vi "Load Calibration Coefficients.vi"() -> (3 "Calibration Coefficients":T1[](array[typedef]) {"Elapsed Time" format="%<%H:%M:%S>t"; "Pump Flow Rate" format="%0d"; "Number of Zeroes" format="%0d"; "V2C" format="%0d"; "C2V" format="%0d"; "duration" format="%<%H:%M:%S>t"; "DAC" format="%03x"; "mI" format="%.3g"; "V_(RA,15mA)" format="%0.4f"; "V_(RA,5mA)" format="%0.4f"; "Chamber Temp" format="%.1f"; "Humidity" format="%.1f"})   [LabVIEW 2016]
uses:
  Controls/Calibration Coefficients.ctl
  Miscellaneous/Globals.vi
panel:
  out "Numeric":i32
  out "size(s)":i32[](array[numeric])
  out "Fini":string
  out "Spreadsheet":string[][](array[string])
  in  "Calfile":path=path "~last_calibration.csv"
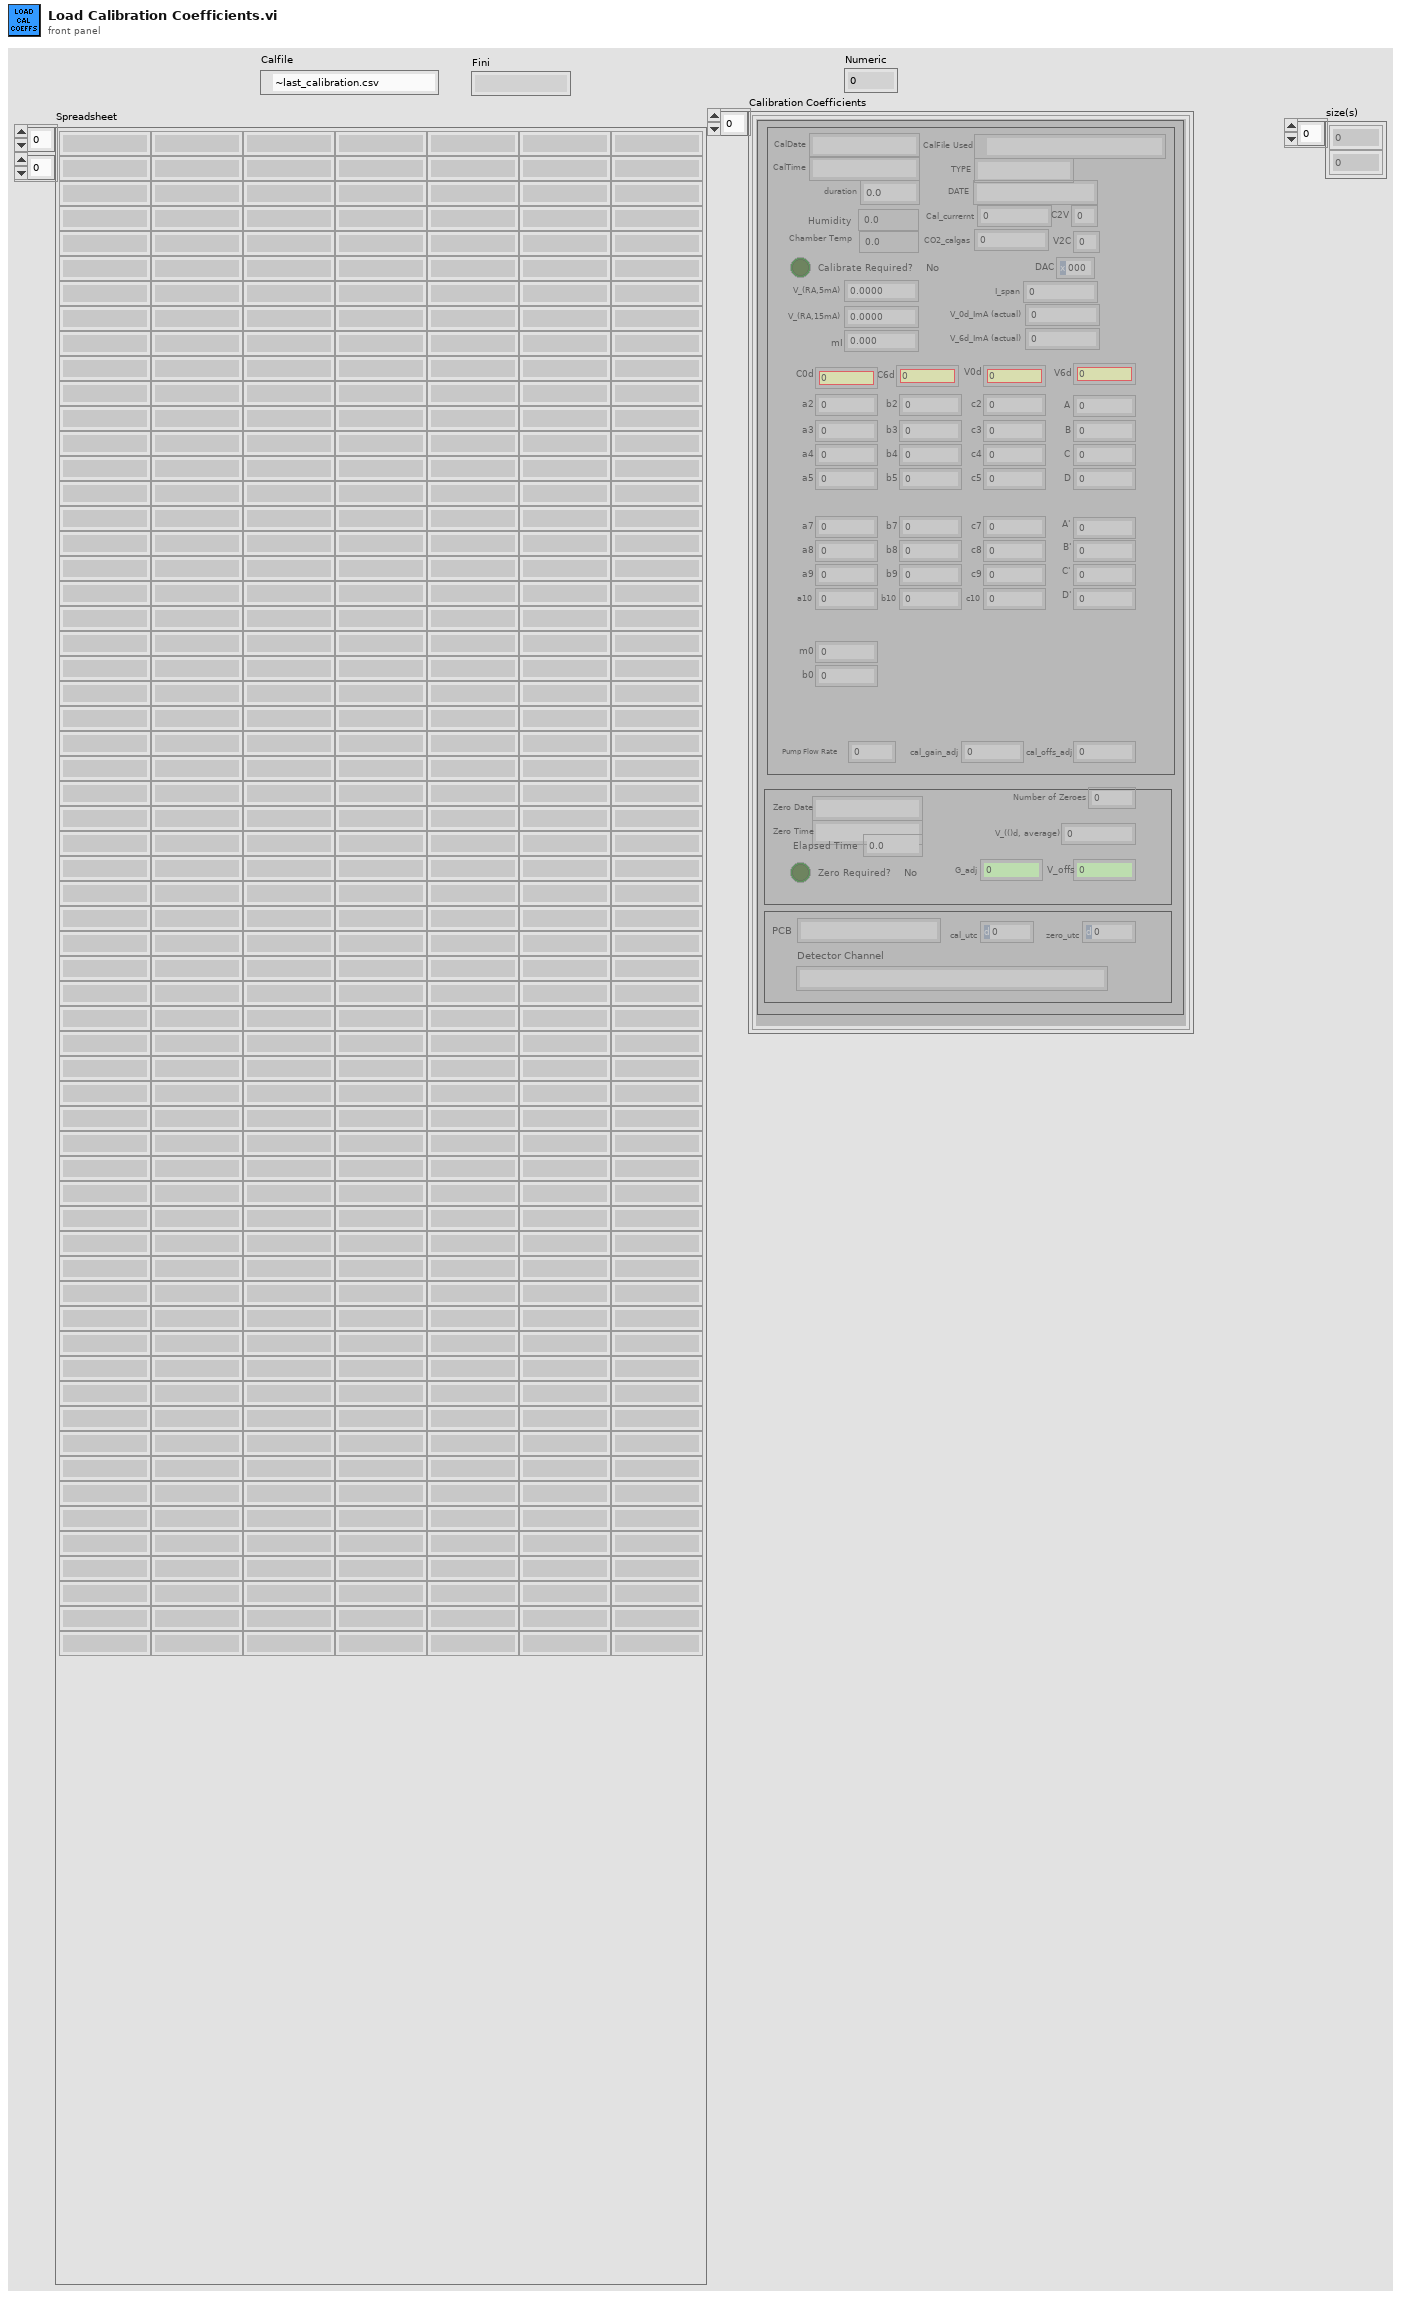
[diagram p1: front panel]
types:
  T1 = typedef "Calibration Coefficients.ctl" = cluster{"CalFile Used":path, "TYPE":string, "DATE":string, "Humidity":sgl, "Chamber Temp":dbl, "CO2_calgas":dbl, "V_(RA,5mA)":dbl, "V_(RA,15mA)":dbl, "mI":dbl, "V_0d_ImA (actual)":dbl, "V_6d_ImA (actual)":dbl, "I_span":dbl, "DAC":u16, "A":dbl, "B":dbl, "C":dbl, "D":dbl, "V6d":dbl, "A'":dbl, "B'":dbl, "C'":dbl, "D'":dbl, "V0d":dbl, "CalDate":string, "CalTime":string, "duration":dbl, "Detector Channel":string, "a2":dbl, "a3":dbl, "a4":dbl, "a5":dbl, "b2":dbl, "c2":dbl, "b3":dbl, "c3":dbl, "b4":dbl, "c4":dbl, "b5":dbl, "c5":dbl, "a7":dbl, "a8":dbl, "a9":dbl, "a10":dbl, "b7":dbl, "b8":dbl, "b9":dbl, "b10":dbl, "c7":dbl, "c8":dbl, "c9":dbl, "c10":dbl, "cal_offs_adj":dbl, "cal_gain_adj":dbl, "C6d":dbl, "C0d":dbl, "Cal_currernt":dbl, "C2V":u16, "V2C":u16, "Zero Date":string, "Zero Time":string, "Number of Zeroes":u16, "V_(()d, average)":dbl, "V_offs ":dbl, "G_adj":dbl, "Pump Flow Rate":u16, "Zero Required? ":bool, "Calibrate Required?":bool, "cal_utc":dbl, "zero_utc":dbl, "Elapsed Time":dbl, "PCB":string, "m0":dbl, "b0":dbl}
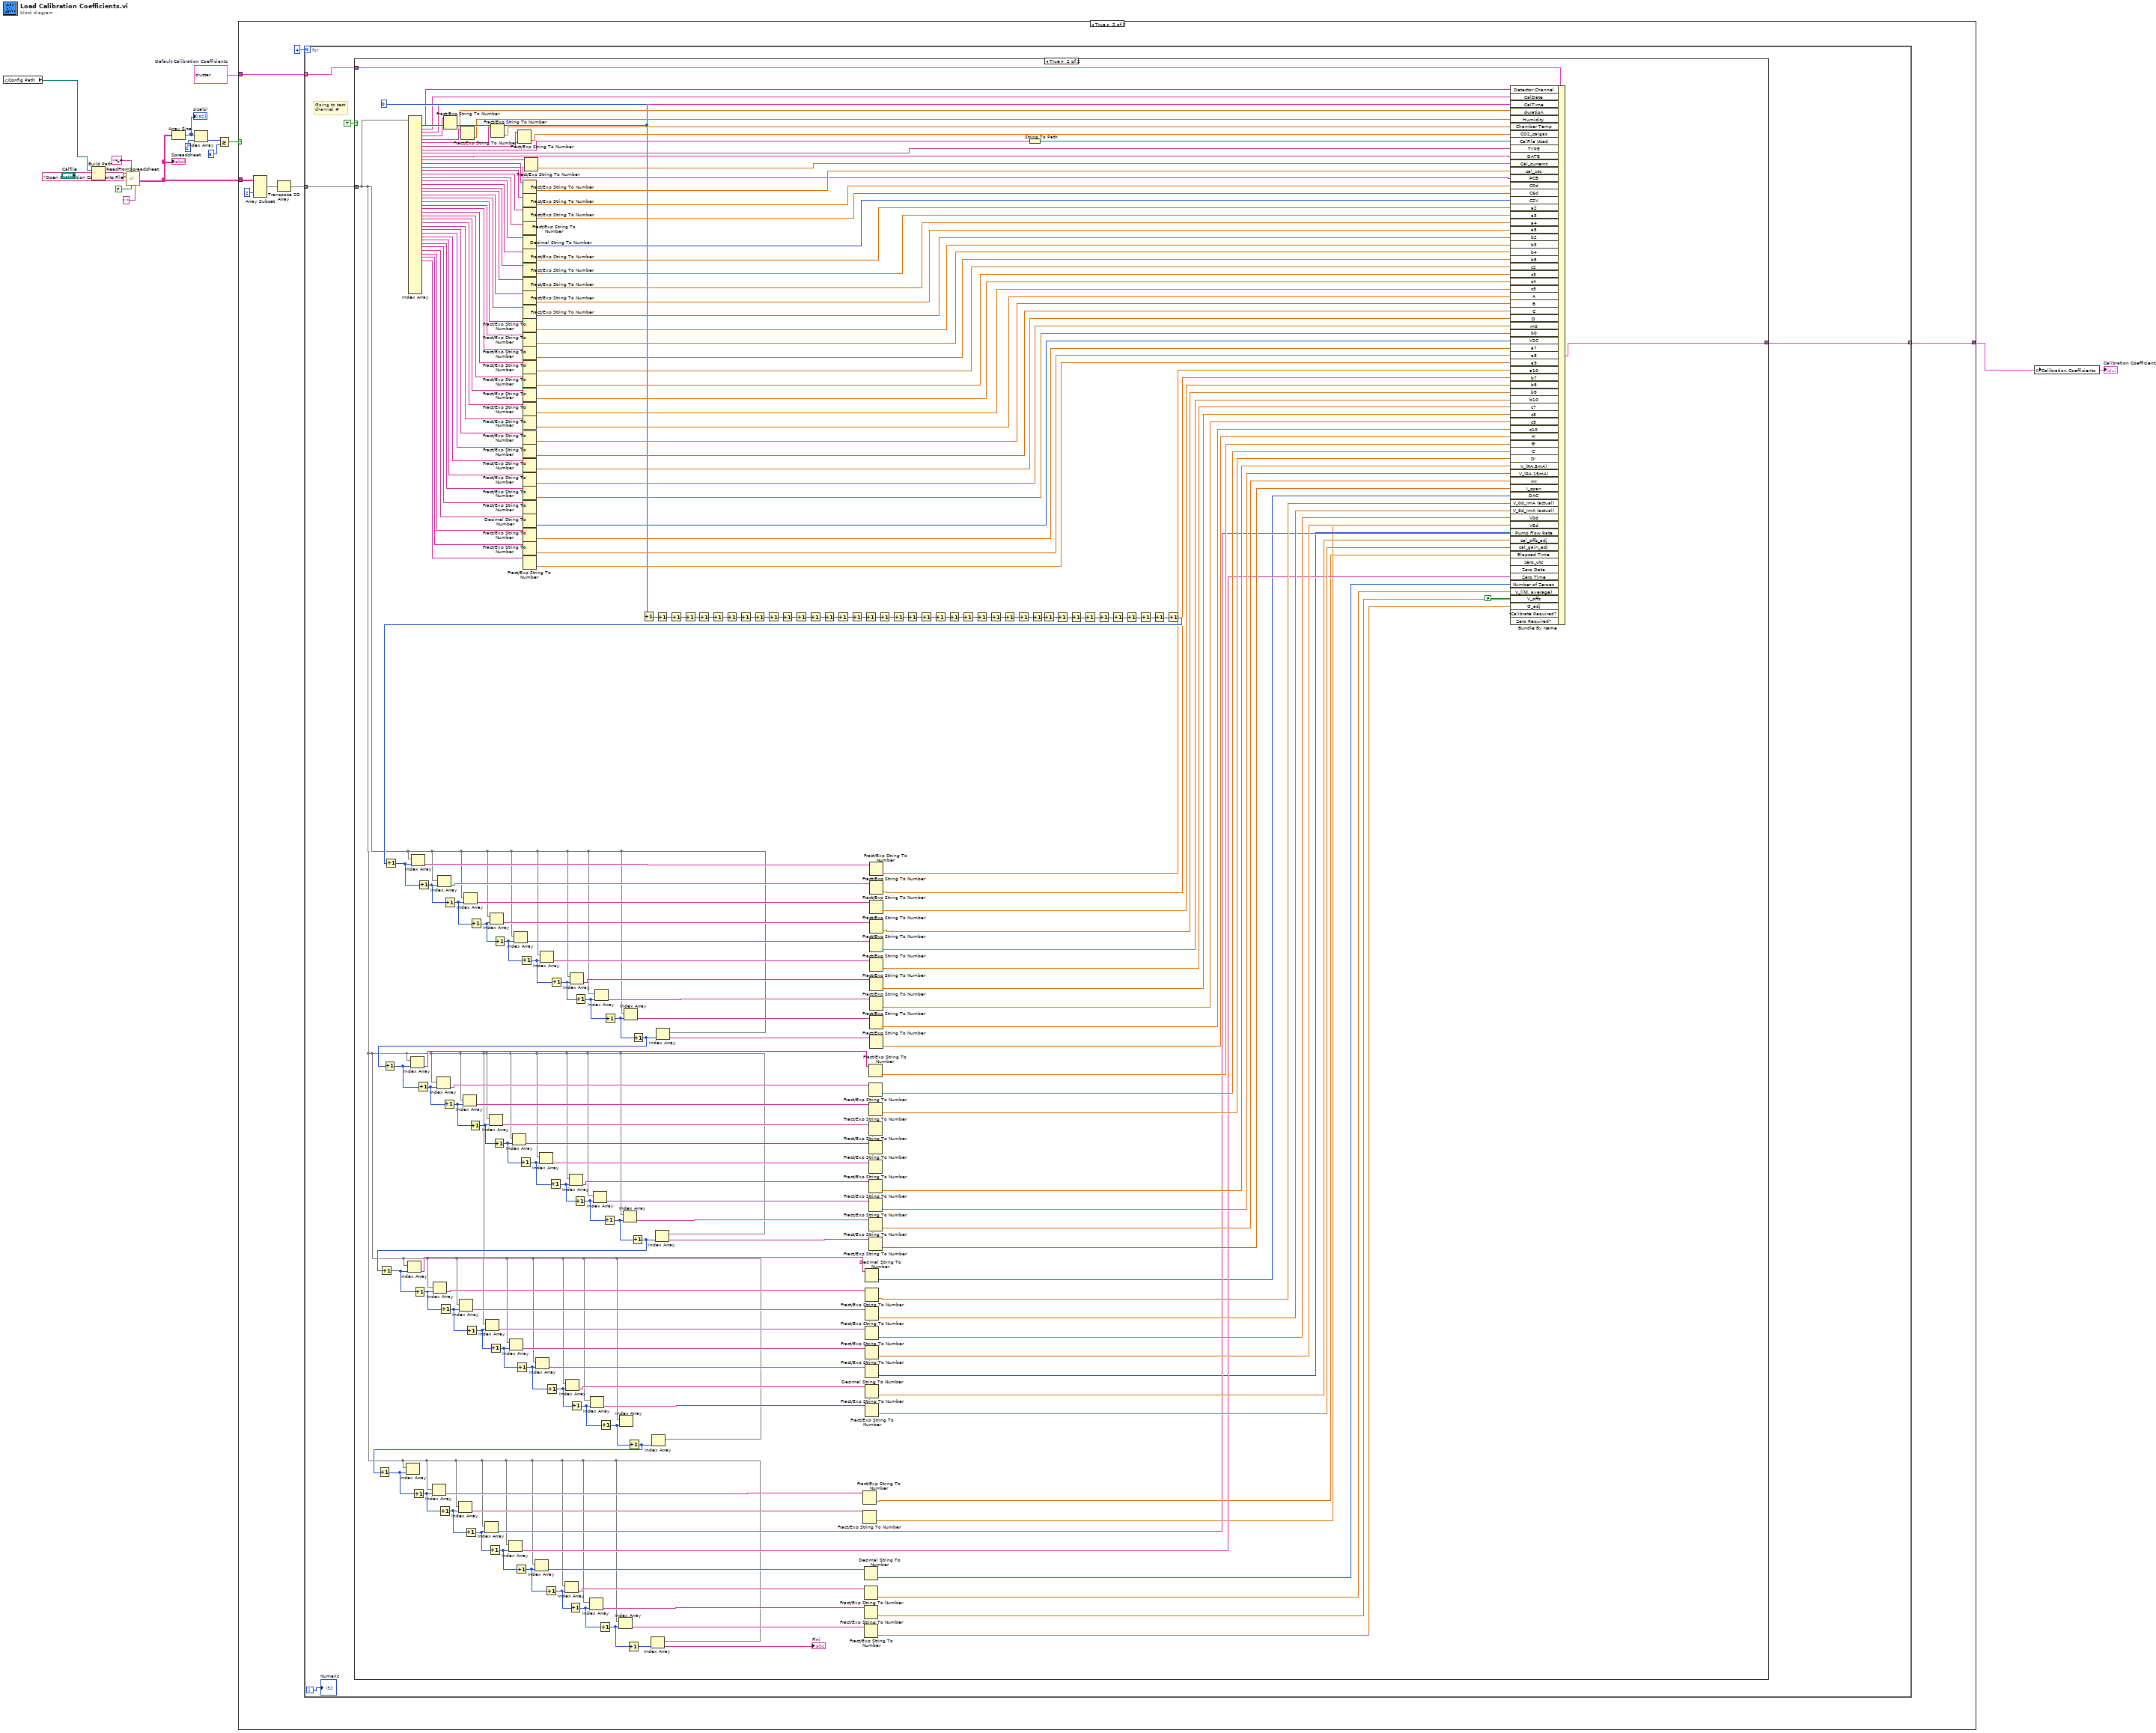
[diagram p0: block diagram]
diagram:
  w4 = T1[] [{"CalFile Used"=path "C:/Users/Bench2/Dropbox/PAHS Public/AK Temp/Coefficients/AE_coefficents.CSV", "TYPE"="CalCoeff", "DATE"="[04-07-15]&[04-16-15]", "Humidity"=114.68759, "Chamber Temp"=20.714597, "CO2_calgas"=6.0, "V_(RA,5mA)"=0.52354, "V_(RA,15mA)"=1.619069, "mI"=109.552915, "V_0d_ImA (actual)"=1.442862, "V_6d_ImA (actual)"=4.943226, "I_span"=0.0132, "DAC"=126, "A"=0.008886, "B"=-0.182423, "C"=1.620623, "D"=1.075523, "V6d"=6.151482, "A'"=0.029909, "B'"=-0.16462, "C'"=0.985378, "D'"=-0.927836, "V0d"=1.188075, "CalDate"="6/2/2015", "CalTime"="4:50:14 PM", "duration"=214.0, "Detector Channel"="1", "a2"=1.6e-05, "a3"=-0.000231, "a4"=0.000552, "a5"=-0.001022, "b2"=-0.001316, "c2"=0.029462, "b3"=0.021946, "c3"=-0.537873, "b4"=-0.098377, "c4"=3.421543, "b5"=0.038523, "c5"=0.716135, "a7"=2e-05, "a8"=0.000362, "a9"=0.00167, "a10"=-0.001204, "b7"=-0.000903, "b8"=-0.00141, "b9"=-0.087565, "b10"=0.06077, "c7"=0.040003, "c8"=-0.29086, "c9"=2.082505, "c10"=-1.670048, "cal_offs_adj"=0.254787, "cal_gain_adj"=1.004082, "C6d"=5.866368, "C0d"=0.060659, "Cal_currernt"=8.0, "C2V"=4, "V2C"=4, "Zero Date"="6/2/2015", "Zero Time"="4:50:18 PM", "Number of Zeroes"=0, "V_(()d, average)"=1.442862, "V_offs "=0.254787, "G_adj"=1.004082, "Pump Flow Rate"=150, "Zero Required? "=FALSE, "Calibrate Required?"=FALSE, "cal_utc"=3516105014.176389, "zero_utc"=3516105018.776652, "Elapsed Time"=0.0, "PCB"="", "m0"=nan, "b0"=nan}, {"CalFile Used"=path "C:/Users/Bench2/Dropbox/PAHS Public/AK Temp/Coefficients/AE_coefficents.CSV", "TYPE"="CalCoeff", "DATE"="[04-07-15]&[04-16-15]", "Humidity"=114.68759, "Chamber Temp"=20.714597, "CO2_calgas"=6.0, "V_(RA,5mA)"=0.52354, "V_(RA,15mA)"=1.619069, "mI"=109.552915, "V_0d_ImA (actual)"=1.442862, "V_6d_ImA (actual)"=4.943226, "I_span"=0.0132, "DAC"=126, "A"=0.008886, "B"=-0.182423, "C"=1.620623, "D"=1.075523, "V6d"=6.151482, "A'"=0.029909, "B'"=-0.16462, "C'"=0.985378, "D'"=-0.927836, "V0d"=1.188075, "CalDate"="6/2/2015", "CalTime"="4:50:14 PM", "duration"=214.0, "Detector Channel"="2", "a2"=1.6e-05, "a3"=-0.000231, "a4"=0.000552, "a5"=-0.001022, "b2"=-0.001316, "c2"=0.029462, "b3"=0.021946, "c3"=-0.537873, "b4"=-0.098377, "c4"=3.421543, "b5"=0.038523, "c5"=0.716135, "a7"=2e-05, "a8"=0.000362, "a9"=0.00167, "a10"=-0.001204, "b7"=-0.000903, "b8"=-0.00141, "b9"=-0.087565, "b10"=0.06077, "c7"=0.040003, "c8"=-0.29086, "c9"=2.082505, "c10"=-1.670048, "cal_offs_adj"=0.254787, "cal_gain_adj"=1.004082, "C6d"=5.866368, "C0d"=0.060659, "Cal_currernt"=8.0, "C2V"=4, "V2C"=4, "Zero Date"="6/2/2015", "Zero Time"="4:50:18 PM", "Number of Zeroes"=0, "V_(()d, average)"=1.442862, "V_offs "=0.254787, "G_adj"=1.004082, "Pump Flow Rate"=150, "Zero Required? "=FALSE, "Calibrate Required?"=FALSE, "cal_utc"=3516105014.176389, "zero_utc"=3516105018.776652, "Elapsed Time"=0.0, "PCB"="", "m0"=nan, "b0"=nan}, {"CalFile Used"=path "C:/Users/Bench2/Dropbox/PAHS Public/AK Temp/Coefficients/AE_coefficents.CSV", "TYPE"="CalCoeff", "DATE"="[04-07-15]&[04-16-15]", "Humidity"=114.68759, "Chamber Temp"=20.714597, "CO2_calgas"=6.0, "V_(RA,5mA)"=0.52354, "V_(RA,15mA)"=1.619069, "mI"=109.552915, "V_0d_ImA (actual)"=1.442862, "V_6d_ImA (actual)"=4.943226, "I_span"=0.0132, "DAC"=126, "A"=0.008886, "B"=-0.182423, "C"=1.620623, "D"=1.075523, "V6d"=6.151482, "A'"=0.029909, "B'"=-0.16462, "C'"=0.985378, "D'"=-0.927836, "V0d"=1.188075, "CalDate"="6/2/2015", "CalTime"="4:50:14 PM", "duration"=214.0, "Detector Channel"="3", "a2"=1.6e-05, "a3"=-0.000231, "a4"=0.000552, "a5"=-0.001022, "b2"=-0.001316, "c2"=0.029462, "b3"=0.021946, "c3"=-0.537873, "b4"=-0.098377, "c4"=3.421543, "b5"=0.038523, "c5"=0.716135, "a7"=2e-05, "a8"=0.000362, "a9"=0.00167, "a10"=-0.001204, "b7"=-0.000903, "b8"=-0.00141, "b9"=-0.087565, "b10"=0.06077, "c7"=0.040003, "c8"=-0.29086, "c9"=2.082505, "c10"=-1.670048, "cal_offs_adj"=0.254787, "cal_gain_adj"=1.004082, "C6d"=5.866368, "C0d"=0.060659, "Cal_currernt"=8.0, "C2V"=4, "V2C"=4, "Zero Date"="6/2/2015", "Zero Time"="4:50:18 PM", "Number of Zeroes"=0, "V_(()d, average)"=1.442862, "V_offs "=0.254787, "G_adj"=1.004082, "Pump Flow Rate"=150, "Zero Required? "=FALSE, "Calibrate Required?"=FALSE, "cal_utc"=3516105014.176389, "zero_utc"=3516105018.776652, "Elapsed Time"=0.0, "PCB"="", "m0"=nan, "b0"=nan}, {"CalFile Used"=path "C:/Users/Bench2/Dropbox/PAHS Public/AK Temp/Coefficients/AE_coefficents.CSV", "TYPE"="CalCoeff", "DATE"="[04-07-15]&[04-16-15]", "Humidity"=114.68759, "Chamber Temp"=20.714597, "CO2_calgas"=6.0, "V_(RA,5mA)"=0.52354, "V_(RA,15mA)"=1.619069, "mI"=109.552915, "V_0d_ImA (actual)"=1.442862, "V_6d_ImA (actual)"=4.943226, "I_span"=0.0132, "DAC"=126, "A"=0.008886, "B"=-0.182423, "C"=1.620623, "D"=1.075523, "V6d"=6.151482, "A'"=0.029909, "B'"=-0.16462, "C'"=0.985378, "D'"=-0.927836, "V0d"=1.188075, "CalDate"="6/2/2015", "CalTime"="4:50:14 PM", "duration"=214.0, "Detector Channel"="4", "a2"=1.6e-05, "a3"=-0.000231, "a4"=0.000552, "a5"=-0.001022, "b2"=-0.001316, "c2"=0.029462, "b3"=0.021946, "c3"=-0.537873, "b4"=-0.098377, "c4"=3.421543, "b5"=0.038523, "c5"=0.716135, "a7"=2e-05, "a8"=0.000362, "a9"=0.00167, "a10"=-0.001204, "b7"=-0.000903, "b8"=-0.00141, "b9"=-0.087565, "b10"=0.06077, "c7"=0.040003, "c8"=-0.29086, "c9"=2.082505, "c10"=-1.670048, "cal_offs_adj"=0.254787, "cal_gain_adj"=1.004082, "C6d"=5.866368, "C0d"=0.060659, "Cal_currernt"=8.0, "C2V"=4, "V2C"=4, "Zero Date"="6/2/2015", "Zero Time"="4:50:18 PM", "Number of Zeroes"=0, "V_(()d, average)"=1.442862, "V_offs "=0.254787, "G_adj"=1.004082, "Pump Flow Rate"=150, "Zero Required? "=FALSE, "Calibrate Required?"=FALSE, "cal_utc"=3516105014.176389, "zero_utc"=3516105018.776652, "Elapsed Time"=0.0, "PCB"="", "m0"=nan, "b0"=nan}]  # Default Calibration Coefficients
  n1 = global read "Globals.vi" "Config Path"() -> (w3:path)
  n2 = Build Path(base path=w3, name or relative path="Calfile") -> (appended path=w11:path)
  n3 = call "ReadFromSpreadsheet.vi"("delimiter (\\t)"="," ("delimiter (\\t)"), "transpose (no:F)"=FALSE, "format (%d)"="%f", "File Prompt"="Open Calibration Coefficients File", "file path"=w11) -> ("text array"=w10:string[][])  [unwired: 2 in, 4 out]
  "Spreadsheet" <- w10
  n4 = Array Size(array=w10) -> (size(s)=w9:i32[])
  "size(s)" <- w9
  n5 = Index Array(array=w9, index=1) -> (element=w6:i32)
  n6 = Greater Or Equal?(x=w6, y=6) -> (x >= y?=w7:bool)
  n7 = case shown="True" w7 {
    tunnel: w10 -> [_ w20]
    tunnel: [w16 w19] -> w2
    tunnel: w4 -> [w16 w18]
    frame False {
    }
    frame True {
      n8 = Array Subset(array=w20, index (col)=2 ("index")) -> (w22:string[][])  [unwired: 3 in]
      n9 = Transpose 2D Array(2D array=w22) -> (transposed array=w21:string[][])
      n10 = for {
        N: 4 -> [_]
        tunnel: w21 -> [w28] mode=indexing
        tunnel: [w27] -> w19 mode=indexing
        tunnel: w18 -> [w26] mode=indexing
        i -> [w24]
        # "Going to test\nchannel #"
        n11 = case shown="True" TRUE {
          tunnel: w28 -> [_ w74]
          tunnel: [w29 w73] -> w27
          tunnel: w26 -> [w29 w72]
          frame False {
          }
          frame True {
            w82 = FALSE
            w253 = 0 ("disabled index (col)")
            n12 = Index Array(array=w74, index #1=w253) -> (element #1=w231:string, element #2=w68:string, element #3=w67:string, element #4=w66:string, element #5=w65:string, element #6=w64:string, element #7=w63:string, element #8=w62:string, element #9=w61:string, element #10=w60:string, element #11=w59:string, element #12=w58:string, element #13=w57:string, element #14=w56:string, element #15=w55:string, element #16=w54:string, element #17=w53:string, element #18=w52:string, element #19=w51:string, element #20=w50:string, element #21=w49:string, element #22=w48:string, element #23=w47:string, element #24=w46:string, element #25=w45:string, element #26=w44:string, element #27=w43:string, element #28=w42:string, element #29=w41:string, element #30=w40:string, element #31=w39:string, element #32=w38:string, element #33=w37:string, element #34=w36:string, element #35=w35:string, element #36=w34:string, element #37=w33:string, element #38=w32:string, element #39=w31:string, element #40=w30:string)  [unwired: 48 in, 9 out]
            n13 = Fract/Exp String To Number(string=w66) -> (number=w236:dbl)  [unwired: 3 in, 1 out]
            n14 = Fract/Exp String To Number(string=w65) -> (number=w234:dbl)  [unwired: 3 in, 1 out]
            n15 = Fract/Exp String To Number(string=w64) -> (number=w233:dbl)  [unwired: 3 in, 1 out]
            n16 = Fract/Exp String To Number(string=w63) -> (number=w232:dbl)  [unwired: 3 in, 1 out]
            n17 = Fract/Exp String To Number(string=w58) -> (number=w81:dbl)  [unwired: 3 in, 1 out]
            n18 = Fract/Exp String To Number(string=w56) -> (number=w76:dbl)  [unwired: 3 in, 1 out]
            n19 = Fract/Exp String To Number(string=w55) -> (number=w75:dbl)  [unwired: 3 in, 1 out]
            n20 = Fract/Exp String To Number(string=w54) -> ()  [unwired: 3 in, 2 out]
            n21 = Decimal String To Number(string=w53) -> (number=w90:i32)  [unwired: 2 in, 1 out]
            n22 = Fract/Exp String To Number(string=w52) -> (number=w228:dbl)  [unwired: 3 in, 1 out]
            n23 = Fract/Exp String To Number(string=w51) -> (number=w227:dbl)  [unwired: 3 in, 1 out]
            n24 = Fract/Exp String To Number(string=w50) -> (number=w226:dbl)  [unwired: 3 in, 1 out]
            n25 = Fract/Exp String To Number(string=w48) -> (number=w136:dbl)  [unwired: 3 in, 1 out]
            n26 = Fract/Exp String To Number(string=w47) -> (number=w135:dbl)  [unwired: 3 in, 1 out]
            n27 = Fract/Exp String To Number(string=w46) -> (number=w134:dbl)  [unwired: 3 in, 1 out]
            n28 = Fract/Exp String To Number(string=w45) -> (number=w133:dbl)  [unwired: 3 in, 1 out]
            n29 = Fract/Exp String To Number(string=w44) -> (number=w132:dbl)  [unwired: 3 in, 1 out]
            n30 = Fract/Exp String To Number(string=w43) -> (number=w131:dbl)  [unwired: 3 in, 1 out]
            n31 = Fract/Exp String To Number(string=w42) -> (number=w130:dbl)  [unwired: 3 in, 1 out]
            n32 = Fract/Exp String To Number(string=w41) -> (number=w129:dbl)  [unwired: 3 in, 1 out]
            n33 = Fract/Exp String To Number(string=w40) -> (number=w128:dbl)  [unwired: 3 in, 1 out]
            n34 = Fract/Exp String To Number(string=w39) -> (number=w127:dbl)  [unwired: 3 in, 1 out]
            n35 = Fract/Exp String To Number(string=w38) -> (number=w126:dbl)  [unwired: 3 in, 1 out]
            n36 = Fract/Exp String To Number(string=w37) -> (number=w125:dbl)  [unwired: 3 in, 1 out]
            n37 = Fract/Exp String To Number(string=w36) -> (number=w70:dbl)  [unwired: 3 in, 1 out]
            n38 = Fract/Exp String To Number(string=w35) -> (number=w69:dbl)  [unwired: 3 in, 1 out]
            n39 = Fract/Exp String To Number(string=w34) -> ()  [unwired: 3 in, 2 out]
            n40 = Decimal String To Number(string=w33) -> (number=w71:i32)  [unwired: 2 in, 1 out]
            n41 = Fract/Exp String To Number(string=w32) -> (number=w124:dbl)  [unwired: 3 in, 1 out]
            n42 = Fract/Exp String To Number(string=w31) -> (number=w123:dbl)  [unwired: 3 in, 1 out]
            n43 = Fract/Exp String To Number(string=w30) -> (number=w122:dbl)  [unwired: 3 in, 1 out]
            n44 = Fract/Exp String To Number(string=w49) -> (number=w137:dbl)  [unwired: 3 in, 1 out]
            n45 = Fract/Exp String To Number(string=w59) -> (number=w229:dbl)  [unwired: 3 in, 1 out]
            n46 = Increment(x=w253) -> (x+1=w246:i32)
            n47 = Increment(x=w246) -> (x+1=w245:i32)
            n48 = Increment(x=w245) -> (x+1=w252:i32)
            n49 = Increment(x=w252) -> (x+1=w251:i32)
            n50 = Increment(x=w251) -> (x+1=w250:i32)
            n51 = Increment(x=w250) -> (x+1=w249:i32)
            n52 = Increment(x=w249) -> (x+1=w248:i32)
            n53 = Increment(x=w248) -> (x+1=w247:i32)
            n54 = Increment(x=w247) -> (x+1=w235:i32)
            n55 = Increment(x=w235) -> (x+1=w89:i32)
            n56 = Increment(x=w89) -> (x+1=w243:i32)
            n57 = Increment(x=w243) -> (x+1=w244:i32)
            n58 = Increment(x=w244) -> (x+1=w237:i32)
            n59 = Increment(x=w237) -> (x+1=w238:i32)
            n60 = Increment(x=w238) -> (x+1=w239:i32)
            n61 = Increment(x=w239) -> (x+1=w240:i32)
            n62 = Increment(x=w240) -> (x+1=w241:i32)
            n63 = Increment(x=w241) -> (x+1=w242:i32)
            n64 = Increment(x=w242) -> (x+1=w217:i32)
            n65 = Increment(x=w217) -> (x+1=w88:i32)
            n66 = Increment(x=w88) -> (x+1=w219:i32)
            n67 = Increment(x=w219) -> (x+1=w218:i32)
            n68 = Increment(x=w218) -> (x+1=w225:i32)
            n69 = Increment(x=w225) -> (x+1=w224:i32)
            n70 = Increment(x=w224) -> (x+1=w223:i32)
            n71 = Increment(x=w223) -> (x+1=w222:i32)
            n72 = Increment(x=w222) -> (x+1=w221:i32)
            n73 = Increment(x=w221) -> (x+1=w220:i32)
            n74 = String To Path(string=w62) -> (path=w230:path)
            n75 = Increment(x=w220) -> (x+1=w208:i32)
            n76 = Increment(x=w208) -> (x+1=w87:i32)
            n77 = Increment(x=w87) -> (x+1=w215:i32)
            n78 = Increment(x=w215) -> (x+1=w216:i32)
            n79 = Increment(x=w216) -> (x+1=w209:i32)
            n80 = Increment(x=w209) -> (x+1=w210:i32)
            n81 = Increment(x=w210) -> (x+1=w211:i32)
            n82 = Increment(x=w211) -> (x+1=w212:i32)
            n83 = Increment(x=w212) -> (x+1=w213:i32)
            n84 = Increment(x=w213) -> (x+1=w214:i32)
            n85 = Increment(x=w214) -> (x+1=w171:i32)
            n86 = Increment(x=w171) -> (x+1=w86:i32)
            n87 = Index Array(array=w74, index=w86) -> (element=w198:string)
            n88 = Increment(x=w86) -> (x+1=w191:i32)
            n89 = Index Array(array=w74, index=w191) -> (element=w199:string)
            n90 = Increment(x=w191) -> (x+1=w190:i32)
            n91 = Index Array(array=w74, index=w190) -> (element=w200:string)
            n92 = Increment(x=w190) -> (x+1=w197:i32)
            n93 = Index Array(array=w74, index=w197) -> (element=w201:string)
            n94 = Increment(x=w197) -> (x+1=w196:i32)
            n95 = Index Array(array=w74, index=w196) -> (element=w202:string)
            n96 = Increment(x=w196) -> (x+1=w195:i32)
            n97 = Index Array(array=w74, index=w195) -> (element=w203:string)
            n98 = Increment(x=w195) -> (x+1=w194:i32)
            n99 = Index Array(array=w74, index=w194) -> (element=w204:string)
            n100 = Increment(x=w194) -> (x+1=w193:i32)
            n101 = Index Array(array=w74, index=w193) -> (element=w205:string)
            n102 = Increment(x=w193) -> (x+1=w192:i32)
            n103 = Index Array(array=w74, index=w192) -> (element=w206:string)
            n104 = Increment(x=w192) -> (x+1=w170:i32)
            n105 = Increment(x=w170) -> (x+1=w83:i32)
            n106 = Index Array(array=w74, index=w83) -> (element=w181:string)
            n107 = Increment(x=w83) -> (x+1=w188:i32)
            n108 = Index Array(array=w74, index=w188) -> (element=w180:string)
            n109 = Increment(x=w188) -> (x+1=w189:i32)
            n110 = Index Array(array=w74, index=w189) -> (element=w179:string)
            n111 = Increment(x=w189) -> (x+1=w182:i32)
            n112 = Index Array(array=w74, index=w182) -> (element=w178:string)
            n113 = Increment(x=w182) -> (x+1=w183:i32)
            n114 = Index Array(array=w74, index=w183) -> (element=w177:string)
            n115 = Increment(x=w183) -> (x+1=w184:i32)
            n116 = Index Array(array=w74, index=w184) -> (element=w176:string)
            n117 = Increment(x=w184) -> (x+1=w185:i32)
            n118 = Index Array(array=w74, index=w185) -> (element=w175:string)
            n119 = Increment(x=w185) -> (x+1=w186:i32)
            n120 = Index Array(array=w74, index=w186) -> (element=w174:string)
            n121 = Increment(x=w186) -> (x+1=w187:i32)
            n122 = Index Array(array=w74, index=w187) -> (element=w173:string)
            n123 = Increment(x=w187) -> (x+1=w138:i32)
            n124 = Increment(x=w138) -> (x+1=w85:i32)
            n125 = Index Array(array=w74, index=w85) -> (element=w146:string)
            n126 = Increment(x=w85) -> (x+1=w153:i32)
            n127 = Index Array(array=w74, index=w153) -> (element=w145:string)
            n128 = Increment(x=w153) -> (x+1=w154:i32)
            n129 = Index Array(array=w74, index=w154) -> (element=w144:string)
            n130 = Increment(x=w154) -> (x+1=w147:i32)
            n131 = Index Array(array=w74, index=w147) -> (element=w143:string)
            n132 = Increment(x=w147) -> (x+1=w148:i32)
            n133 = Index Array(array=w74, index=w148) -> (element=w142:string)
            n134 = Increment(x=w148) -> (x+1=w149:i32)
            n135 = Index Array(array=w74, index=w149) -> (element=w141:string)
            n136 = Increment(x=w149) -> (x+1=w150:i32)
            n137 = Index Array(array=w74, index=w150) -> (element=w140:string)
            n138 = Increment(x=w150) -> (x+1=w151:i32)
            n139 = Index Array(array=w74, index=w151) -> (element=w139:string)
            n140 = Increment(x=w151) -> (x+1=w152:i32)
            n141 = Index Array(array=w74, index=w152) -> ()  [unwired: 1 out]
            n142 = Increment(x=w152) -> (x+1=w169:i32)
            n143 = Increment(x=w169) -> (x+1=w84:i32)
            n144 = Index Array(array=w74, index=w84) -> ()  [unwired: 1 out]
            n145 = Increment(x=w84) -> (x+1=w156:i32)
            n146 = Index Array(array=w74, index=w156) -> (element=w78:string)
            n147 = Increment(x=w156) -> (x+1=w155:i32)
            n148 = Index Array(array=w74, index=w155) -> (element=w80:string)
            n149 = Increment(x=w155) -> (x+1=w162:i32)
            n150 = Index Array(array=w74, index=w162) -> (element=w98:string)
            n151 = Increment(x=w162) -> (x+1=w161:i32)
            n152 = Index Array(array=w74, index=w161) -> (element=w97:string)
            n153 = Increment(x=w161) -> (x+1=w160:i32)
            n154 = Index Array(array=w74, index=w160) -> (element=w164:string)
            n155 = Increment(x=w160) -> (x+1=w159:i32)
            n156 = Index Array(array=w74, index=w159) -> (element=w165:string)
            n157 = Increment(x=w159) -> (x+1=w158:i32)
            n158 = Index Array(array=w74, index=w158) -> (element=w166:string)
            n159 = Increment(x=w158) -> (x+1=w157:i32)
            n160 = Index Array(array=w74, index=w157) -> (element=w167:string)
            n161 = Increment(x=w157) -> (x+1=w163:i32)
            n162 = Index Array(array=w74, index=w163) -> (element=→"Fini":string)
            n163 = Index Array(array=w74, index=w169) -> ()  [unwired: 1 out]
            n164 = Index Array(array=w74, index=w138) -> (element=w172:string)
            n165 = Index Array(array=w74, index=w170) -> (element=w207:string)
            n166 = Fract/Exp String To Number(string=w78) -> (number=w77:dbl)  [unwired: 3 in, 1 out]
            n167 = Fract/Exp String To Number(string=w80) -> (number=w79:dbl)  [unwired: 3 in, 1 out]
            n168 = Decimal String To Number(string=w164) -> (number=w93:i32)  [unwired: 2 in, 1 out]
            n169 = Fract/Exp String To Number(string=w165) -> (number=w96:dbl)  [unwired: 3 in, 1 out]
            n170 = Fract/Exp String To Number(string=w166) -> (number=w95:dbl)  [unwired: 3 in, 1 out]
            n171 = Fract/Exp String To Number(string=w167) -> (number=w94:dbl)  [unwired: 3 in, 1 out]
            n172 = Decimal String To Number(string=w146) -> (number=w91:i32)  [unwired: 2 in, 1 out]
            n173 = Fract/Exp String To Number(string=w145) -> (number=w104:dbl)  [unwired: 3 in, 1 out]
            n174 = Fract/Exp String To Number(string=w144) -> (number=w103:dbl)  [unwired: 3 in, 1 out]
            n175 = Fract/Exp String To Number(string=w143) -> (number=w102:dbl)  [unwired: 3 in, 1 out]
            n176 = Fract/Exp String To Number(string=w142) -> (number=w101:dbl)  [unwired: 3 in, 1 out]
            n177 = Decimal String To Number(string=w141) -> (number=w92:i32)  [unwired: 2 in, 1 out]
            n178 = Fract/Exp String To Number(string=w140) -> (number=w100:dbl)  [unwired: 3 in, 1 out]
            n179 = Fract/Exp String To Number(string=w139) -> (number=w99:dbl)  [unwired: 3 in, 1 out]
            n180 = Fract/Exp String To Number(string=w181) -> (number=w111:dbl)  [unwired: 3 in, 1 out]
            n181 = Fract/Exp String To Number(string=w180) -> (number=w110:dbl)  [unwired: 3 in, 1 out]
            n182 = Fract/Exp String To Number(string=w179) -> (number=w109:dbl)  [unwired: 3 in, 1 out]
            n183 = Fract/Exp String To Number(string=w178) -> ()  [unwired: 3 in, 2 out]
            n184 = Fract/Exp String To Number(string=w177) -> ()  [unwired: 3 in, 2 out]
            n185 = Fract/Exp String To Number(string=w176) -> ()  [unwired: 3 in, 2 out]
            n186 = Fract/Exp String To Number(string=w175) -> (number=w108:dbl)  [unwired: 3 in, 1 out]
            n187 = Fract/Exp String To Number(string=w174) -> (number=w107:dbl)  [unwired: 3 in, 1 out]
            n188 = Fract/Exp String To Number(string=w173) -> (number=w106:dbl)  [unwired: 3 in, 1 out]
            n189 = Fract/Exp String To Number(string=w172) -> (number=w105:dbl)  [unwired: 3 in, 1 out]
            n190 = Fract/Exp String To Number(string=w198) -> (number=w121:dbl)  [unwired: 3 in, 1 out]
            n191 = Fract/Exp String To Number(string=w199) -> (number=w120:dbl)  [unwired: 3 in, 1 out]
            n192 = Fract/Exp String To Number(string=w200) -> (number=w119:dbl)  [unwired: 3 in, 1 out]
            n193 = Fract/Exp String To Number(string=w201) -> (number=w118:dbl)  [unwired: 3 in, 1 out]
            n194 = Fract/Exp String To Number(string=w202) -> (number=w117:dbl)  [unwired: 3 in, 1 out]
            n195 = Fract/Exp String To Number(string=w203) -> (number=w116:dbl)  [unwired: 3 in, 1 out]
            n196 = Fract/Exp String To Number(string=w204) -> (number=w115:dbl)  [unwired: 3 in, 1 out]
            n197 = Fract/Exp String To Number(string=w205) -> (number=w114:dbl)  [unwired: 3 in, 1 out]
            n198 = Fract/Exp String To Number(string=w206) -> (number=w113:dbl)  [unwired: 3 in, 1 out]
            n199 = Fract/Exp String To Number(string=w207) -> (number=w112:dbl)  [unwired: 3 in, 1 out]
            n200 = Bundle By Name(cluster=w72, "Detector Channel"=w231, "CalDate"=w68, "CalTime"=w67, "duration"=w236, "Humidity"=w234, "Chamber Temp"=w233, "CO2_calgas"=w232, "CalFile Used"=w230, "TYPE"=w61, "DATE"=w60, "Cal_currernt"=w229, "cal_utc"=w81, "PCB"=w57, "C0d"=w76, "C6d"=w75, "C2V"=w90, "a2"=w228, "a3"=w227, "a4"=w226, "a5"=w137, "b2"=w136, "b3"=w135, "b4"=w134, "b5"=w133, "c2"=w132, "c3"=w131, "c4"=w130, "c5"=w129, "A"=w128, "B"=w127, "C"=w126, "D"=w125, "m0"=w70, "b0"=w69, "V2C"=w71, "a7"=w124, "a8"=w123, "a9"=w122, "a10"=w121, "b7"=w120, "b8"=w119, "b9"=w118, "b10"=w117, "c7"=w116, "c8"=w115, "c9"=w114, "c10"=w113, "A'"=w112, "B'"=w111, "C'"=w110, "D'"=w109, "V_(RA,5mA)"=w108, "V_(RA,15mA)"=w107, "mI"=w106, "I_span"=w105, "DAC"=w91, "V_0d_ImA (actual)"=w104, "V_6d_ImA (actual)"=w103, "V0d"=w102, "V6d"=w101, "Pump Flow Rate"=w92, "cal_offs_adj"=w100, "cal_gain_adj"=w99, "Elapsed Time"=w77, "zero_utc"=w79, "Zero Date"=w98, "Zero Time"=w97, "Number of Zeroes"=w93, "V_(()d, average)"=w96, "V_offs"=w95, "G_adj"=w94, "Calibrate Required?"=w82, "Zero Required?"=w82) -> (w73:T1)
          }
        }
        "Numeric" <- w24
      }
    }
  }
  "Calibration Coefficients" <- w2
  n201 = global write "Globals.vi" "Calibration Coefficients"(w2) -> ()
